vi "UsrProfiles-Source-Last used profile section.vi"() -> (0 "Last Used Profile section name":string)   [LabVIEW 2017]
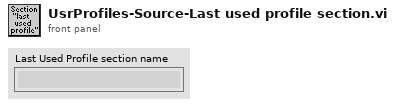
[diagram p1: front panel]
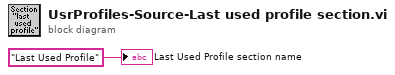
[diagram p0: block diagram]
diagram:
  "Last Used Profile section name" <- "Last Used Profile" ("section")
